vi "Bridge tubo.vi"() -> (2 "tespTUBO":string, 3 "cmdTUBO":string)   [LabVIEW 2018]
uses:
  TCSPD-OPD/TCSPD LV2018/TCSPD 1.0.25.3/Global_Telescopio.vi
panel:
  in  "stop":bool
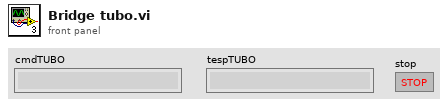
[diagram p1: front panel]
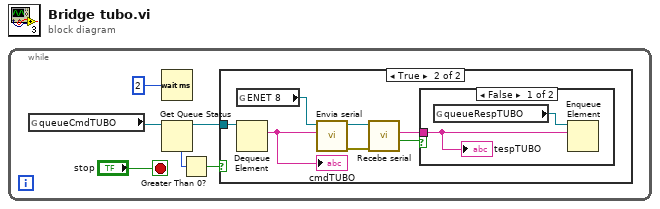
[diagram p0: block diagram]
diagram:
  n1 = while {
    stop <- "stop" stop-if-true
    n2 = global read "Global_Telescopio.vi" "queueCmdTUBO"() -> (w2:refnum<queue>)
    n3 = Wait (ms)(milliseconds to wait=u32 2) -> ()  [unwired: 1 out]
    n4 = Get Queue Status(queue=w2) -> (queue out=w5:refnum<queue>, # elements in queue=w4:i32)  [unwired: 2 in, 6 out]
    n5 = Greater Than 0?(x=w4) -> (x > 0?=w3:bool)
    n6 = case shown="True" w3 {
      tunnel: w5 -> [_ w7]
      frame False {
      }
      frame True {
        n7 = global read "Global_Telescopio.vi" "ENET 8"() -> (w9:refnum<visa-resource-name>)
        n8 = Dequeue Element(queue=w7) -> (element=w8:string)  [unwired: 2 in, 3 out]
        "cmdTUBO" <- w8
        n9 = call "Envia serial.vi"("String a ser Enviado"=w8, "LNA VISA session (for class)"=w9) -> ("error out"=w10:errorcluster, "LNA VISA session saida"=w11:refnum<visa-resource-name>)  [unwired: 6 in, 2 out]
        n10 = call "Recebe serial.vi"("error in (no error)"=w10, "LNA VISA resource name"=w11) -> ("timeout"=w13:bool, "String Lida"=w12:string)  [unwired: 6 in, 2 out]
        n11 = case shown="False" w13 {
          tunnel: w12 -> [w14 _]
          frame False {
            n12 = global read "Global_Telescopio.vi" "queueRespTUBO"() -> (w15:refnum<queue>)
            n13 = Enqueue Element(queue=w15, element=w14) -> ()  [unwired: 2 in, 3 out]
            "tespTUBO" <- w14
          }
          frame True {
          }
        }
      }
    }
  }
